vi "SW_TO_CMD.vi"() -> ()   [LabVIEW 2018]
panel:
  out "Close":string
  out "Open":string
  in  "64 SW OUT":bool[](array[boolean])
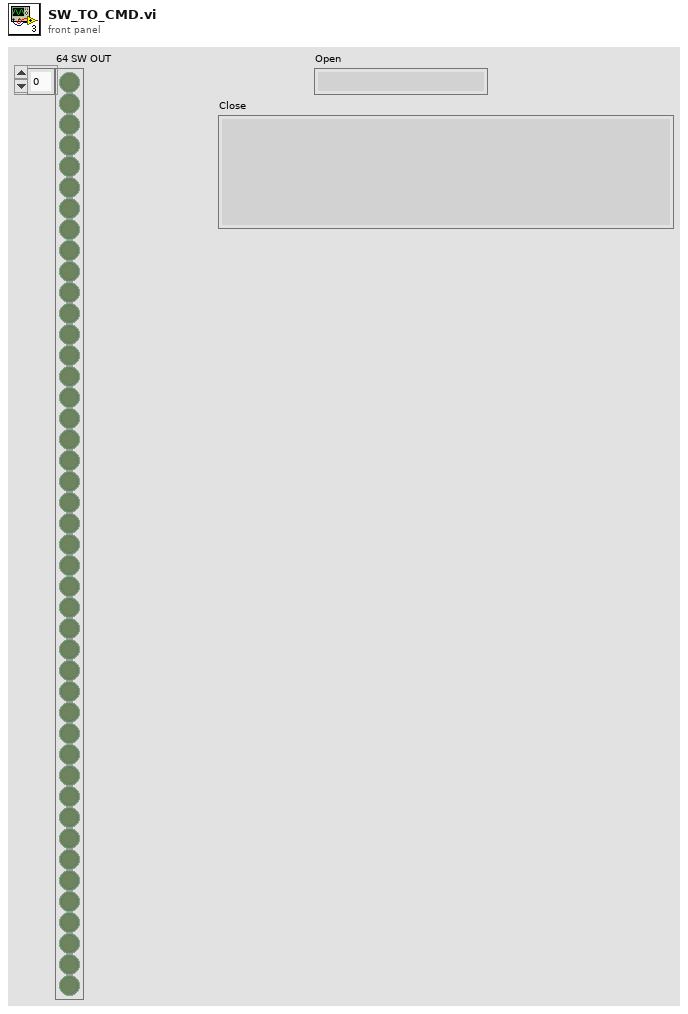
[diagram p1: front panel]
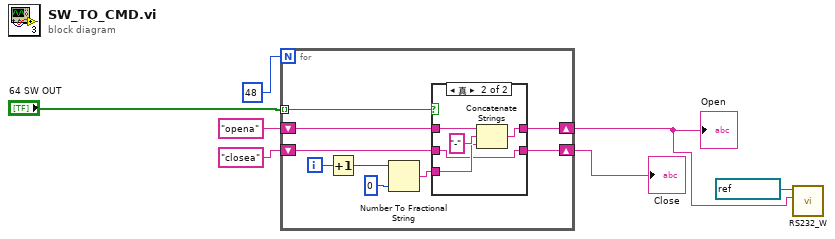
[diagram p0: block diagram]
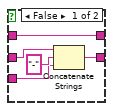
[diagram p2: hidden frame]
diagram:
  n1 = for {
    N: 48 -> [_]
    tunnel: "64 SW OUT" -> [w11] mode=indexing
    shift-right: [w12] -> w1
    shift-left: "opena" -> [w10]
    shift-right: [w8] -> w2
    shift-left: "closea" -> [w9]
    i -> [w16]
    n2 = Increment(x=w16) -> (x+1=w15:i32)
    n3 = Number To Fractional String(number=w15, precision (6)=i16 0 ("精度(6)")) -> (F-format string=w13:string)  [unwired: 2 in]
    n4 = case shown="真" w11 {
      tunnel: w13 -> [w20 w24]
      tunnel: [w18 w26] -> w12
      tunnel: w10 -> [w18 w22]
      tunnel: w9 -> [w17 w23]
      tunnel: [w19 w23] -> w8
      frame False {
        n5 = Concatenate Strings(w17, "-", w20) -> (w19:string)
      }
      frame True {
        n6 = Concatenate Strings(w22, "-", w24) -> (w26:string)
      }
    }
  }
  "Open" <- w1
  "Close" <- w2
  n7 = call "RS232_W.vi"("CMD"=w1, "VISA资源名称"=refnum<visa-resource-name> "COM6" ("VISA资源名称 2")) -> ()  [unwired: 8 in, 2 out]
